vi "Formula_Node_Ejercicio.vi"() -> ()   [LabVIEW 2020]
panel:
  out "Grafico de un Circulo":cluster{dbl[], dbl[]}(graph)
  out "Waveform Graph":dbl[](graph)
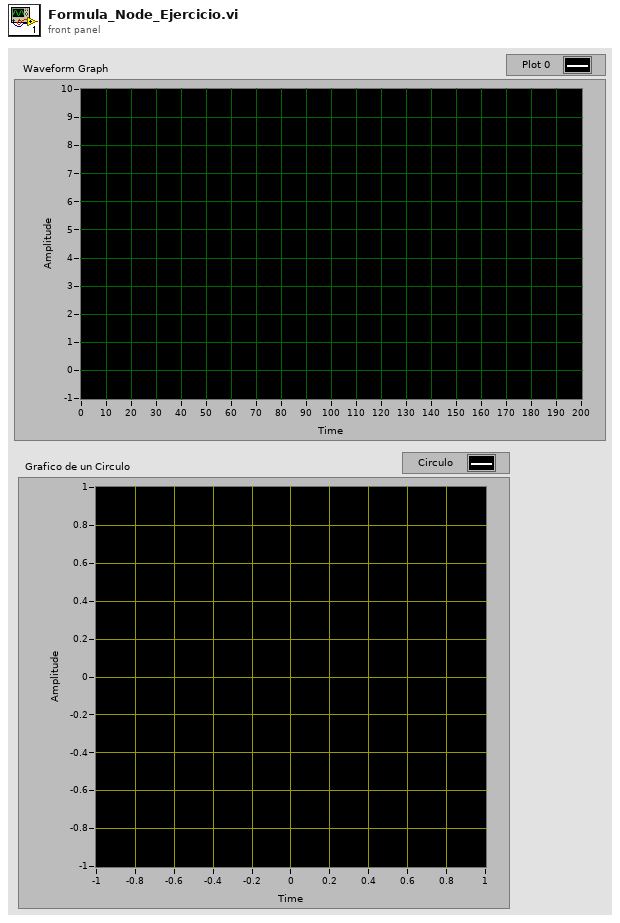
[diagram p1: front panel]
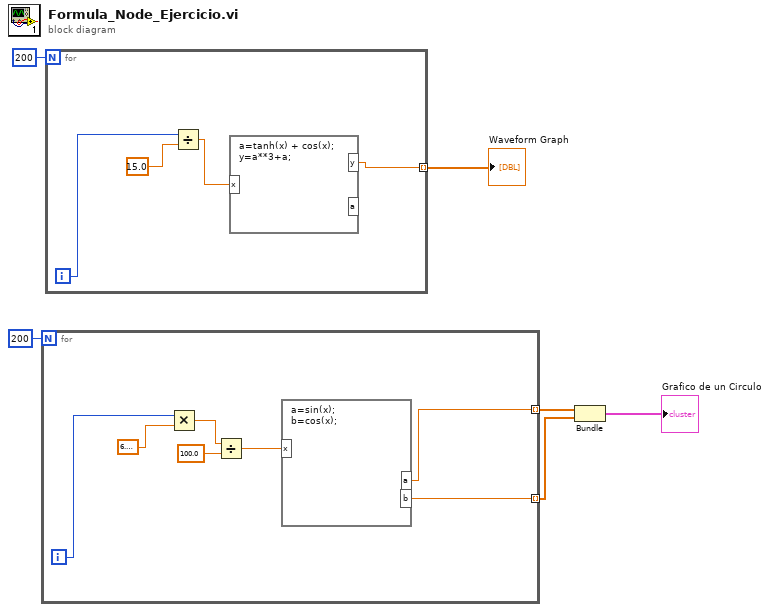
[diagram p0: block diagram]
diagram:
  n1 = for {
    N: 200 -> [_]
    tunnel: [w8] -> w3 mode=indexing
    tunnel: [w7] -> w2 mode=indexing
    i -> [w9]
    n2 = Multiply(x=w9, y=6.283185307179586) -> (x*y=w12:dbl)
    n3 = Divide(x=w12, y=100.0) -> (x/y=w10:dbl)
    n4 = formula code="a=sin(x);\nb=cos(x);"("x"=w10) -> ("b"=w7:dbl, "a"=w8:dbl)
  }
  n5 = for {
    N: 200 -> [_]
    tunnel: [w14] -> w5 mode=indexing
    i -> [w17]
    n6 = Divide(x=w17, y=15.0) -> (x/y=w15:dbl)
    n7 = formula code="a=tanh(x) + cos(x);\ny=a**3+a;"("x"=w15) -> ("y"=w14:dbl)  [unwired: 1 out]
  }
  "Waveform Graph" <- w5
  n8 = Bundle(w3, w2) -> (→"Grafico de un Circulo":cluster{dbl[], dbl[]})  [unwired: 1 in]
